vi "NPSV FIFO test.vi"() -> ()   [LabVIEW 2019]
uses:
  Reverse Polarity.ctl
  Forward Polarity.ctl
  Motion Controller Slot.ctl
  Stepper Output Configuration.ctl
  Axis Select.ctl
  MsgTypeDef.ctl
  DataDef.ctl
  <vilib>/NI/Modbus Library/API/Modbus API.lvclass
  <vilib>/WPC Systems Ltd/GECO Driver/Lib/GECOBase/GECO_Driver Class/GECO_Driver.lvclass
  <vilib>/WPC Systems Ltd/GECO Driver/Lib/GECOMotion/GECOMotion/_typedefine/Axis Select.ctl
  <vilib>/WPC Systems Ltd/GECO Driver/Lib/GECOBase/GECO_Driver Class/Motion/_typedefine/GECO_Stepper Output Configuration.ctl
  <vilib>/WPC Systems Ltd/GECO Driver/Lib/GECOBase/GECO_Driver Class/Motion/_typedefine/GECO_Motion Operation Mode.ctl
  <vilib>/WPC Systems Ltd/GECO Driver/Lib/GECOBase/GECO_Driver Class/GECO_SlotName.ctl
  <vilib>/WPC Systems Ltd/GECO Driver/Lib/GECOBase/GECO_Driver Class/Motion/_typedefine/GECO_ActiveHighLow.ctl
  <vilib>/WPC Systems Ltd/GECO Driver/Lib/GECOMotion/GECOMotion/GECO Motion.lvclass
  GyroDef.ctl
  <vilib>/Instr/_visa.llb/VISA Configure Serial Port (Instr).vi
panel:
  out "error IO 2":errorcluster
  out "error IO":errorcluster
  out "實際角度":cluster{"A":dbl, "B":dbl}={"A"=-3.299667554384925, "B"=3.520332445615068}
  out "實際角度Chart":cluster{"X":dbl, "Y":dbl}(graph)={"X"=-3.299667554384925, "Y"=3.520332445615068} caption="Waveform Chart - dark"
  out "Gyro\nPeriod":u32
  in  "Main Setting Tab":T1(tab)
  in  "TimerON":bool
  in  "Timer(ms)":i32=1
  in  "Serial Port":refnum<visa-resource-name>="COM3"
  in  "TCP slave port":u32=1
  in  "baud rate":u32=115200
  in  "Byte bits":u32=8
  in  "Modbus Address Starting":u32
  in  "Modbus Number of Inputs":u32=10000
  in  "Resource Name":tag="rio://192.168.0.224/RIO0"
  in  "Servo on":bool
  in  "Axis Select":T2
  in  "Stepper Output Configuration":T3=enum."CW/CCW(Two Pulse)"
  in  "Forward Enable?":bool=TRUE
  in  "Reverse Enable?":bool=TRUE
  in  "Motion Operation Mode":T4(ring)=enum."Velocity"
  in  "Forward Polarity":T5
  in  "Reverse Polarity":T6
  in  "Motion Controller Slot":T7
  in  "Target Position (0)":dbl=10000.0
  in  "Acceleration (100000)":u32=300000
  in  "Velocity (10000)":dbl=100000.0
  in  "Deacceleration (100000)":u32=300000
  in  "PID gains setting Tab":enum32{"Axis 1", "Axis 2", "Axis 3"}(tab)
  in  "PID gains":T8={"proportional gain (Kc)"=0.75, "integral time (Ti, min)"=0.01, "derivative time (Td, min)"=0.0} {"derivative time (Td, min)" format="%#_3f"; "integral time (Ti, min)" format="%#_3f"; "proportional gain (Kc)" format="%#_3f"}
  in  "PID gains 2":T8={"proportional gain (Kc)"=0.75, "integral time (Ti, min)"=0.01, "derivative time (Td, min)"=0.0} {"derivative time (Td, min)" format="%#_3f"; "integral time (Ti, min)" format="%#_3f"; "proportional gain (Kc)" format="%#_3f"}
  in  "PID gains 3":T8={"proportional gain (Kc)"=0.75, "integral time (Ti, min)"=0.01, "derivative time (Td, min)"=0.0} {"derivative time (Td, min)" format="%#_3f"; "integral time (Ti, min)" format="%#_3f"; "proportional gain (Kc)" format="%#_3f"}
  in  "ZABStop":bool
  in  "B":i32
  in  "A":i32
  in  "Z":i32=50
  in  "ZAB Start":bool
  in  "Move Setting":T9
  out "Axis 1":T10
  out "Axis 2":T10
  out "Axis 3":T10
  out "RT error out":errorcluster
  out "Program Period":u32
  out "RT Program Period":u32
  in  "ServoButtonControl":T11
  in  "Connect":bool
  in  "Close":bool
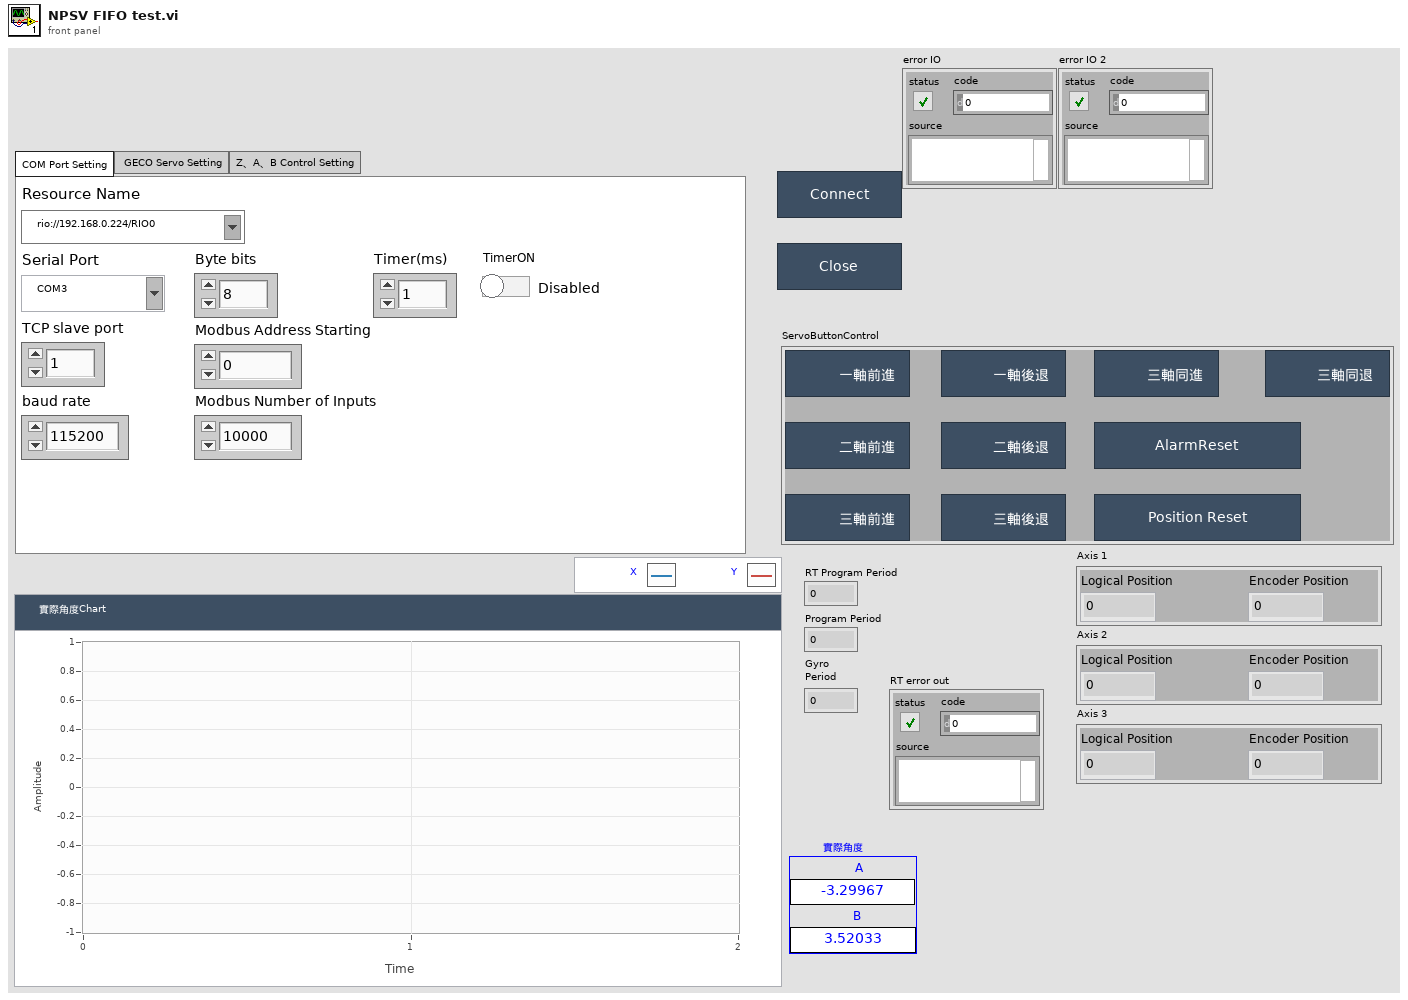
[diagram p1: front panel]
types:
  T1 = enum32{"COM Port Setting", " GECO Servo Setting", "Z、A、B Control Setting"}
  T2 = typedef "Axis Select.ctl" = enum16{"Axis 1", "Axis 2", "Axis 3", "Axis 4"}
  T3 = typedef "Stepper Output Configuration.ctl" = enum16{"Step/Dir(One Pulse)", "CW/CCW(Two Pulse)"}
  T4 = enum16{"Absolute Position", "Relative Position", "Velocity"}
  T5 = typedef "Forward Polarity.ctl" = enum16{"Active High", "Active Low"}
  T6 = typedef "Reverse Polarity.ctl" = enum16{"Active High", "Active Low"}
  T7 = typedef "Motion Controller Slot.ctl" = enum16{"C1", "C2", "C3", "C4"}
  T8 = cluster{"proportional gain (Kc)":dbl, "integral time (Ti, min)":dbl, "derivative time (Td, min)":dbl}
  T9 = typedef "軌跡設定.ctl" = u16
  T10 = cluster{"Encoder Position":i32, "Logical Position":i32}
  T11 = cluster{"三軸同退":bool, "三軸同進":bool, "三軸後退":bool, "三軸前進":bool, "二軸後退":bool, "二軸前進":bool, "一軸後退":bool, "一軸前進":bool, "Reset Encoder Position":bool, "AlarmReset":bool}
  T12 = typedef "GyroDef.ctl" = cluster{"Byte bits":u16, "baud rate":u32, "實際角度":cluster{"A":dbl, "B":dbl}, "COM Port":refnum<visa-resource-name>, "Save Path":refnum<file>}
  T13 = typedef "DataDef.ctl" = cluster{"address starting":u16, "狀態":enum16{"初始化", "讀取", "寫入", "停止"}, "理想角度":cluster{"A":dbl, "B":dbl}, "register values":i16[], "Modbus COM":refnum<class "Modbus API.lvclass">, "TCP slave port":u16, " baud rate":u32, "Byte bits":u16, "ServoButtonControl":cluster{"三軸同退":bool, "三軸同進":bool, "三軸後退":bool, "三軸前進":bool, "二軸後退":bool, "二軸前進":bool, "一軸後退":bool, "一軸前進":bool}, "Serial Number":string, "GECO_Driver out":refnum<class "GECO_Driver.lvclass">, "number of inputs":u16, "ServoSetting":cluster{"Axis Select":T14, "Stepper Output Configuration":T15, "Motion Operation Mode":T16, "Motion Controller Slot":T17, "Singel Axis Move Paramters":cluster{"Motion Operation Mode":T16, "Target Position (0)":i32, "Velocity (10000)":i32, "Acceleration (100000)":u32, "Deacceleration (100000)":u32}, "Reverse":cluster{"Reverse Enable":bool, "Reverse Polarity":T18}, "Forward":cluster{"Forward Enable":bool, "Forward Polarity":T18}}, "GECO Motion out":refnum<class "GECO Motion.lvclass">, "Servo on":bool, "Axis 1 Position":cluster{"Encoder Position":i32, "Logical Position":i32}, "Axis 2 Position":cluster{"Encoder Position":i32, "Logical Position":i32}, "Axis 3 Position":cluster{"Encoder Position":i32, "Logical Position":i32}, "PIDSetting":cluster{"Z":i32, "A":i32, "B":i32, "Move Setting":T19, "Axis Pulse":dbl, "Axis Length":dbl, "PID gains ":cluster{"proportional gain (Kc)":dbl, "integral time (Ti, min)":dbl, "derivative time (Td, min)":dbl}}, "resource name":tag, "Save Path":refnum<file>}
  T14 = typedef "GECO Motion.lvclass/Axis Select.ctl" = enum16{"Axis 1", "Axis 2", "Axis 3", "Axis 4"}
  T15 = typedef "GECO_Driver.lvclass/GECO_Stepper Output Configuration.ctl" = enum16{"Step/Dir(One Pulse)", "CW/CCW(Two Pulse)"}
  T16 = typedef "GECO_Driver.lvclass/GECO_Motion Operation Mode.ctl" = enum16{"Absolute Position", "Relative Position", "Velocity"}
  T17 = typedef "GECO_Driver.lvclass/GECO_SlotName.ctl" = enum16{"C1", "C2", "C3", "C4"}
  T18 = typedef "GECO_Driver.lvclass/GECO_ActiveHighLow.ctl" = enum16{"Active High", "Active Low"}
  T19 = typedef "­y¸ñ.ctl" = u16
  T20 = typedef "MsgTypeDef.ctl" = cluster{"CMD":string, "DATA":variant}
  T21 = enum16{"open", "replace", "create", "open or create", "replace or create", "replace or create with confirmation"}
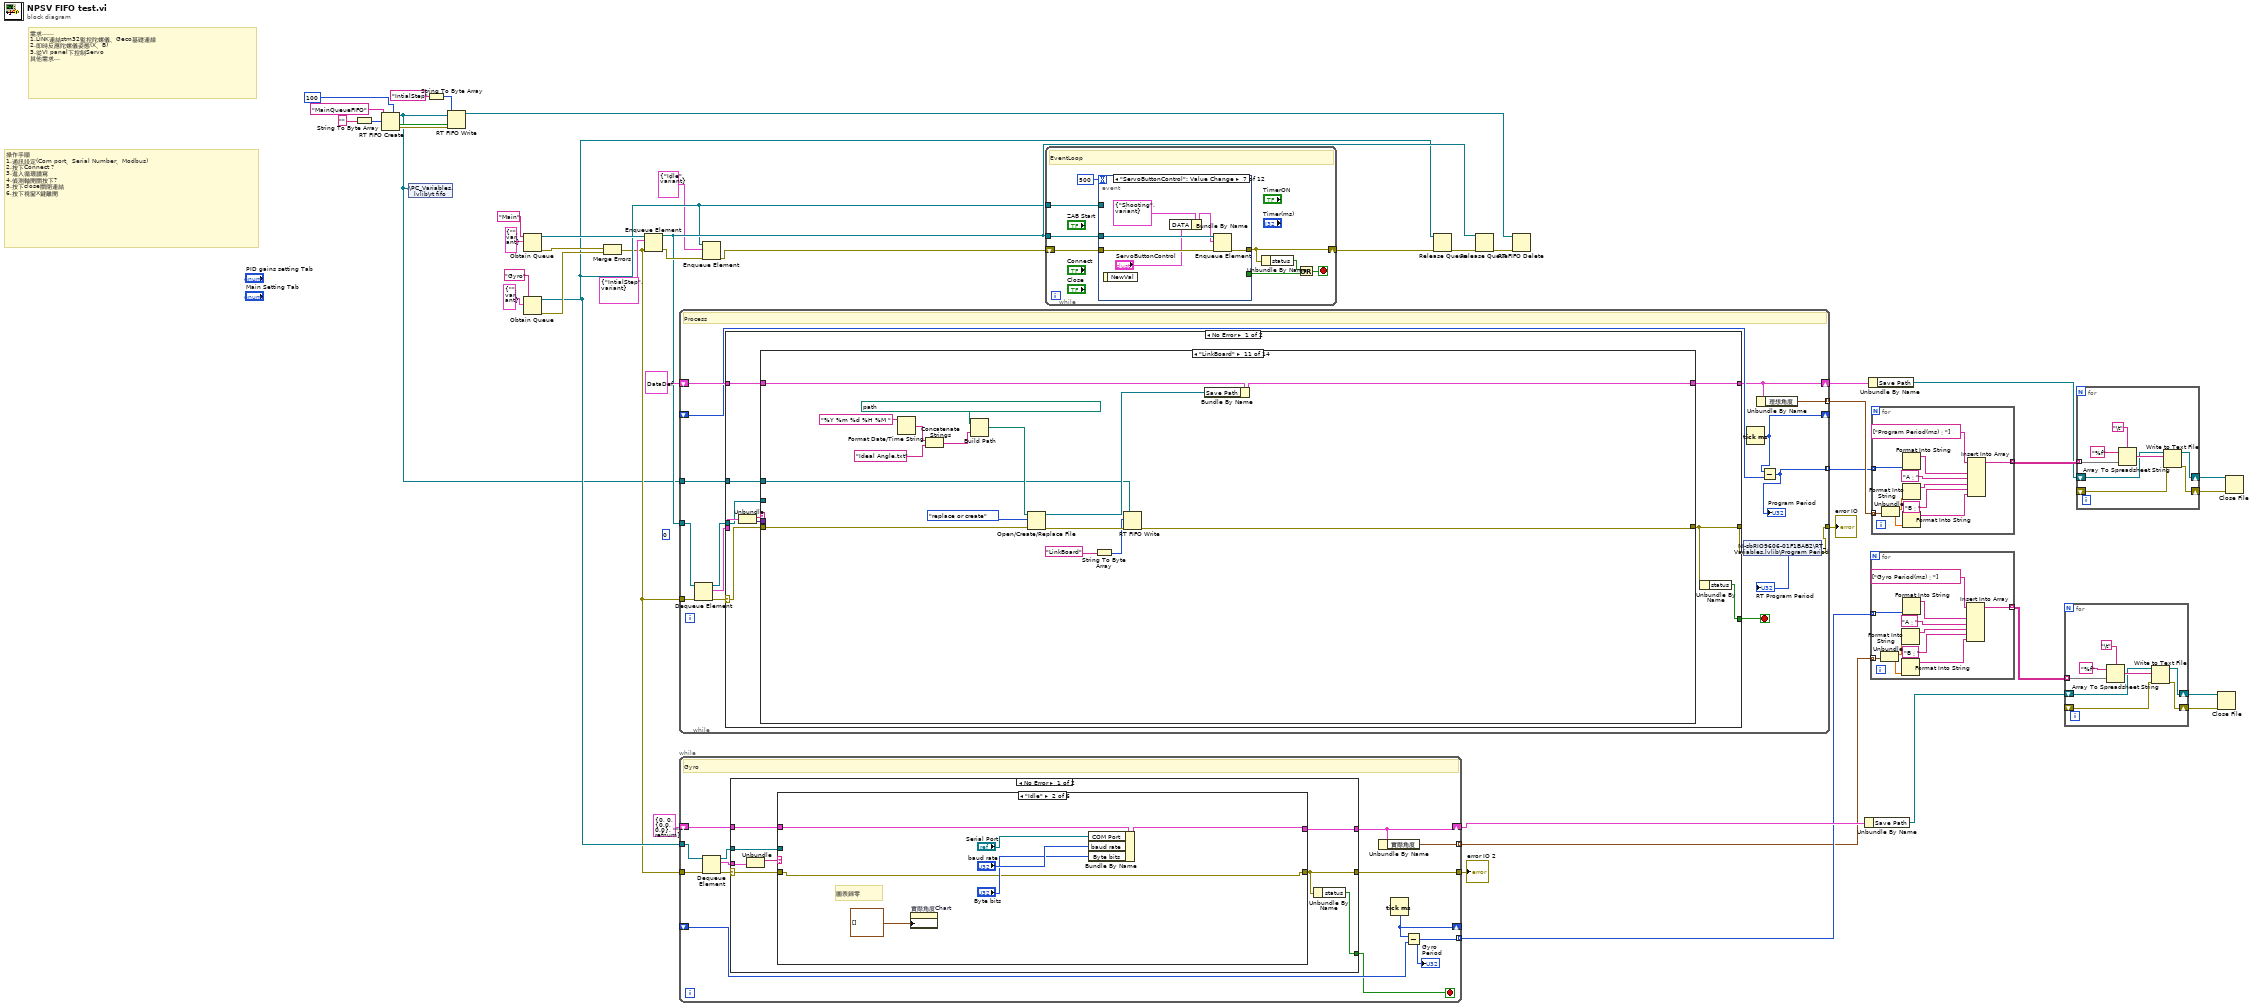
[diagram p0: block diagram]
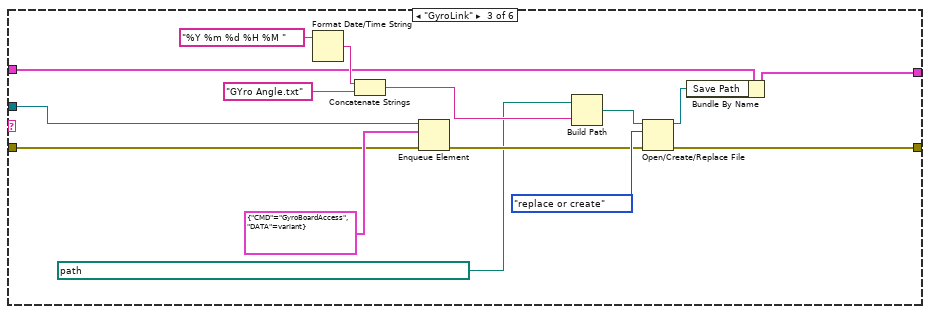
[diagram p3: hidden frame]
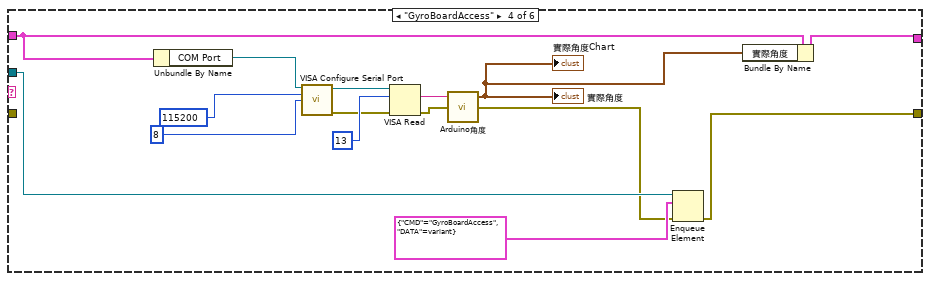
[diagram p4: hidden frame]
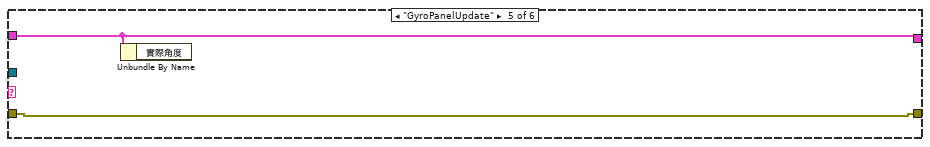
[diagram p5: hidden frame]
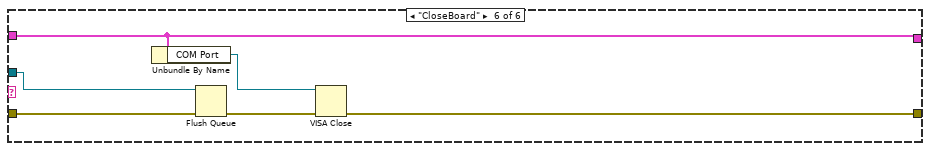
[diagram p6: hidden frame]
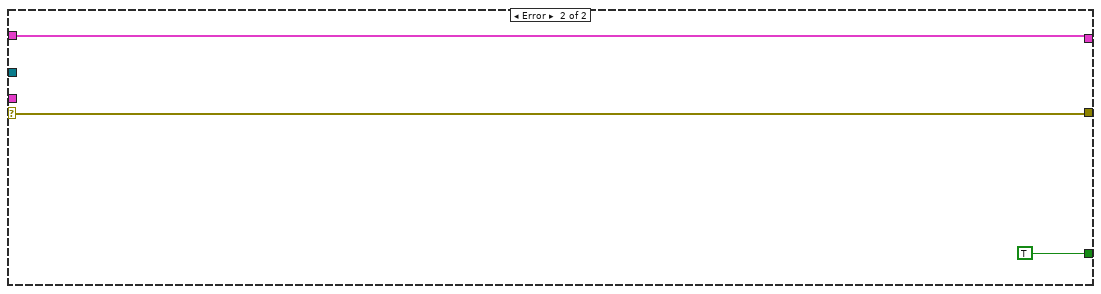
[diagram p7: hidden frame]
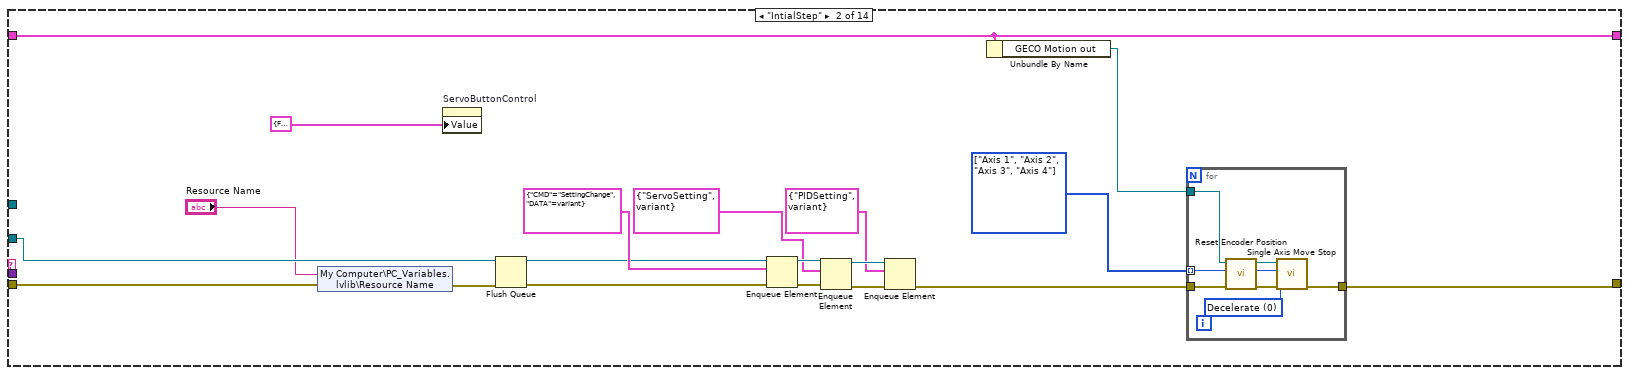
[diagram p9: hidden frame]
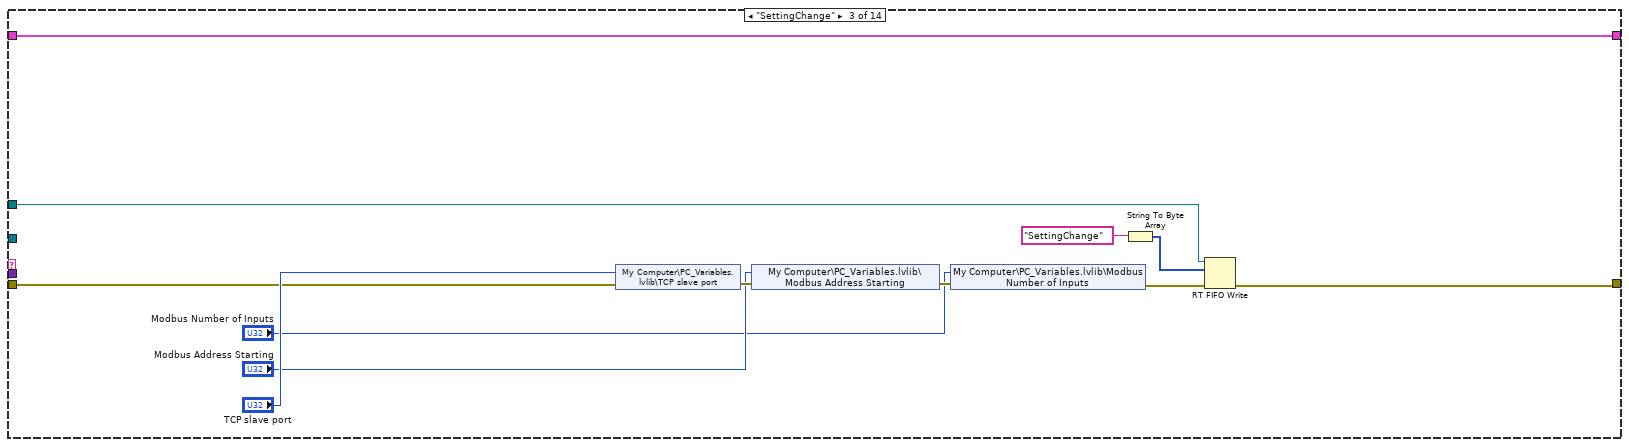
[diagram p10: hidden frame]
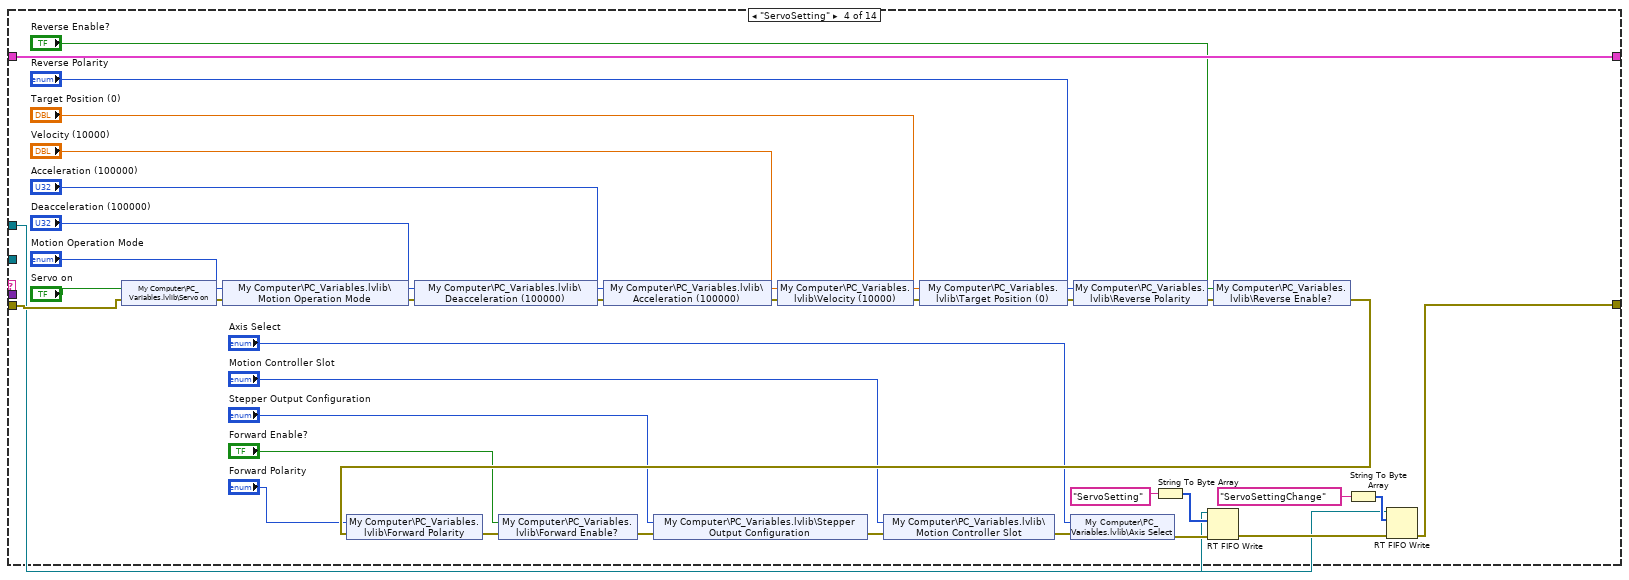
[diagram p11: hidden frame]
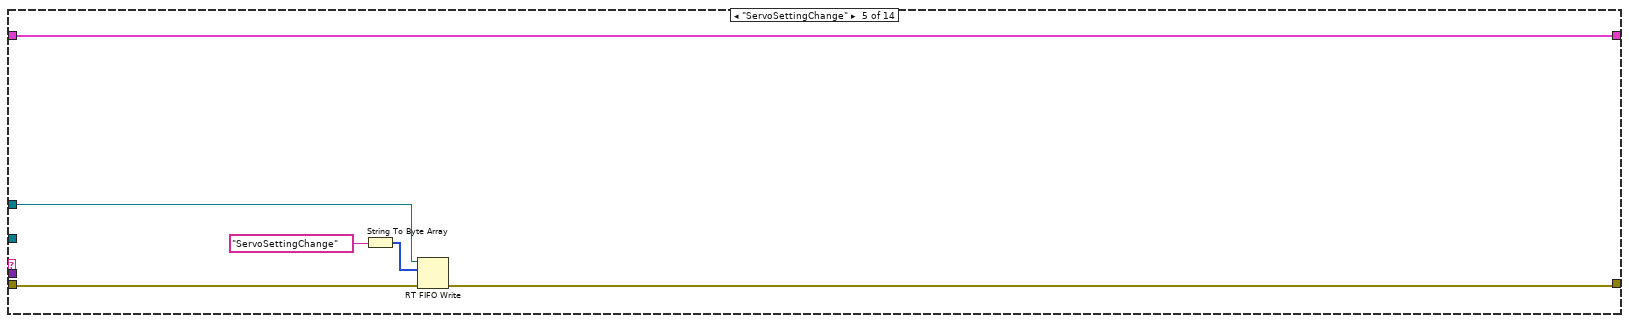
[diagram p12: hidden frame]
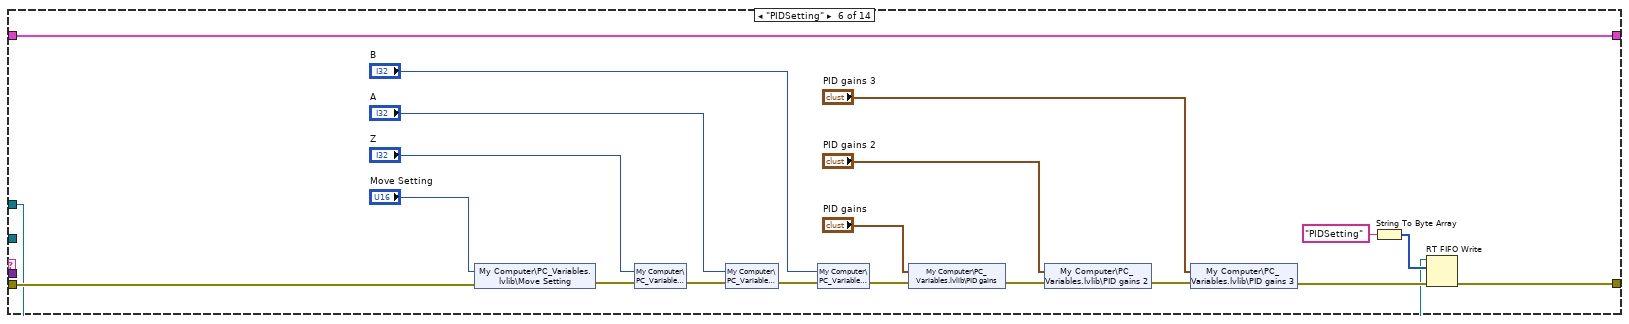
[diagram p13: hidden frame]
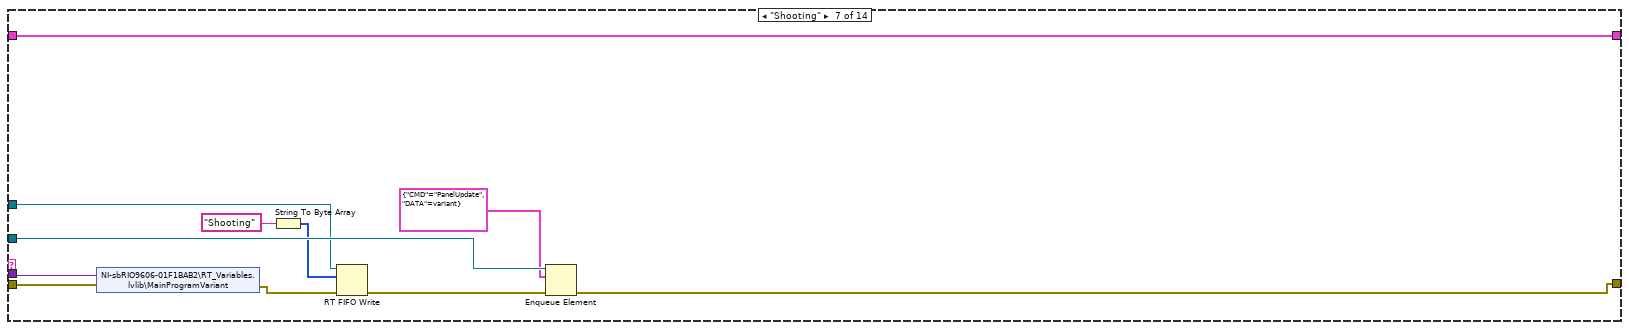
[diagram p14: hidden frame]
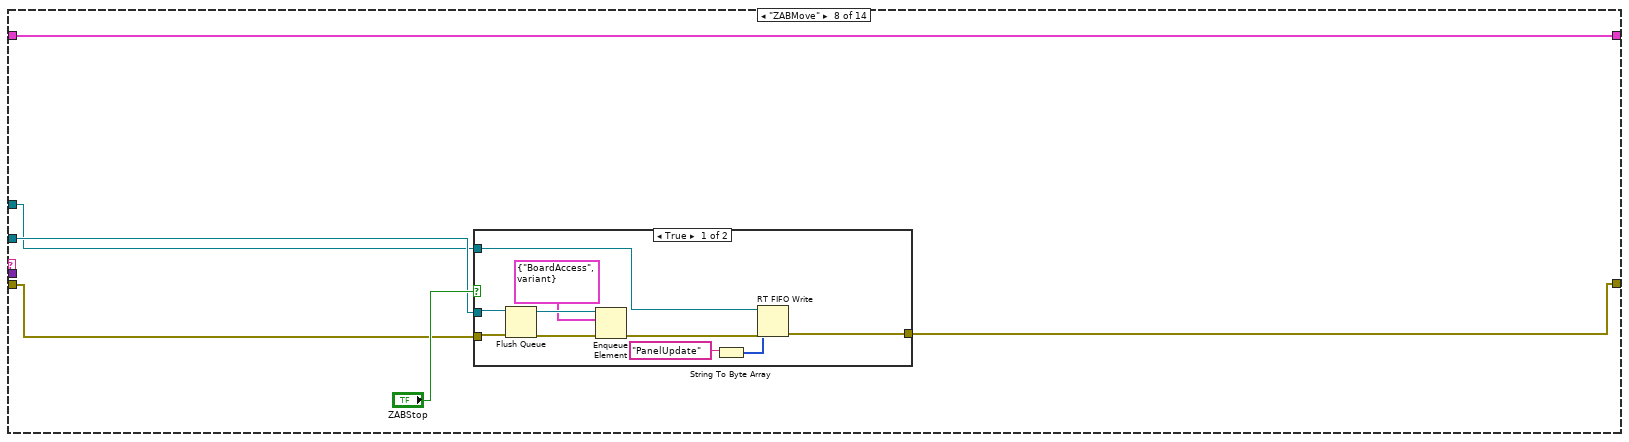
[diagram p15: hidden frame]
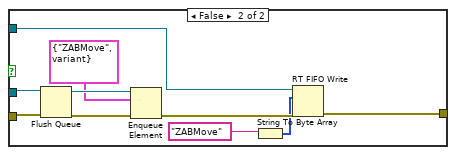
[diagram p16: hidden frame]
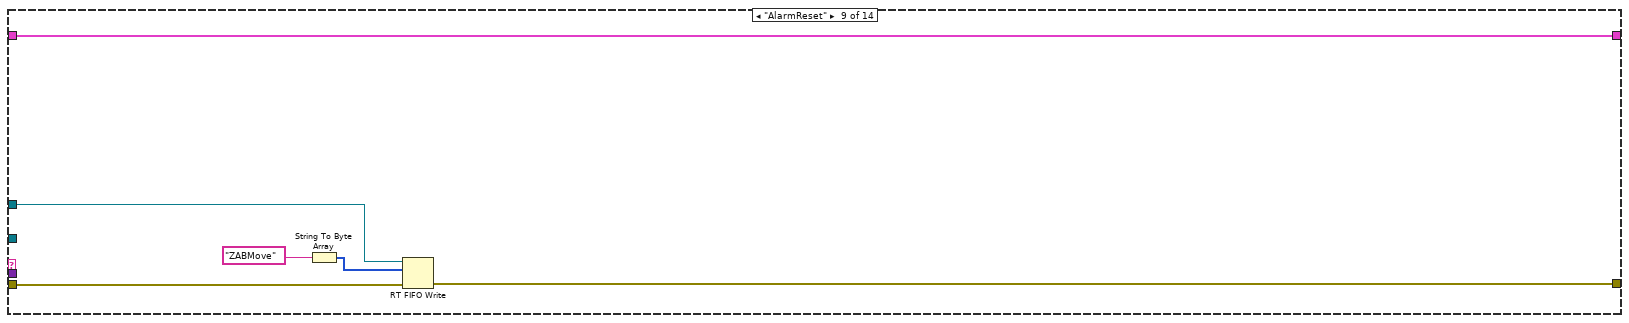
[diagram p17: hidden frame]
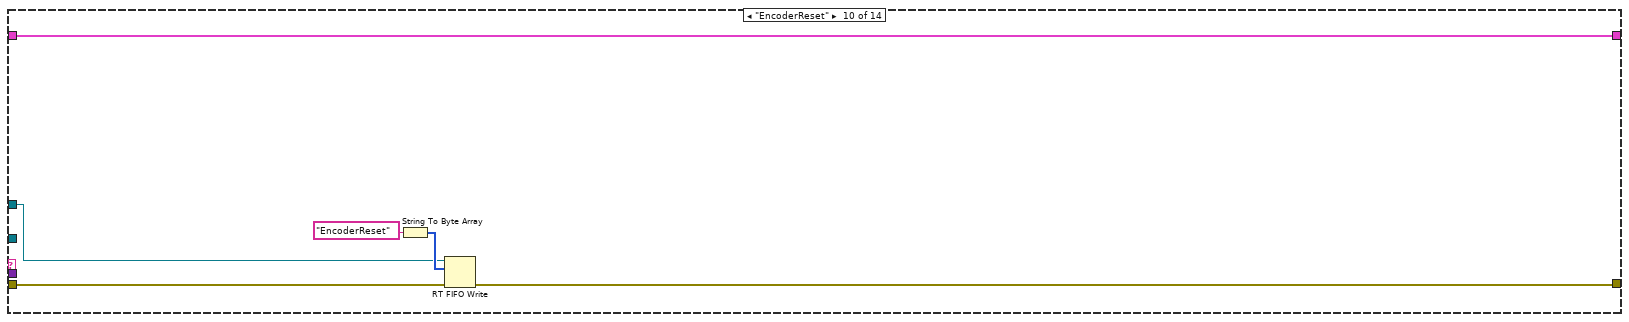
[diagram p18: hidden frame]
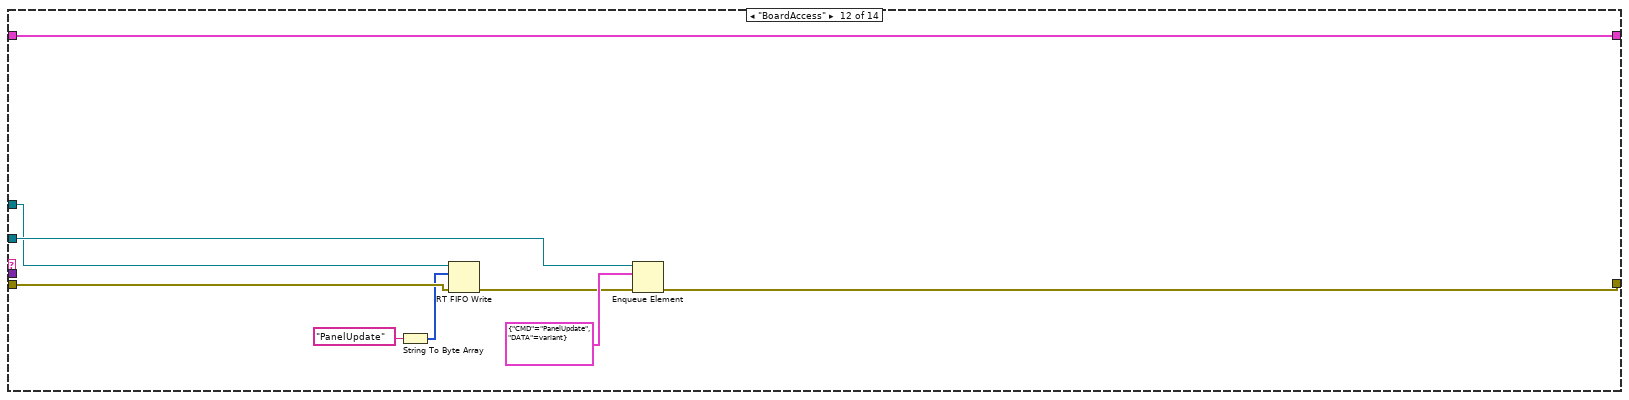
[diagram p19: hidden frame]
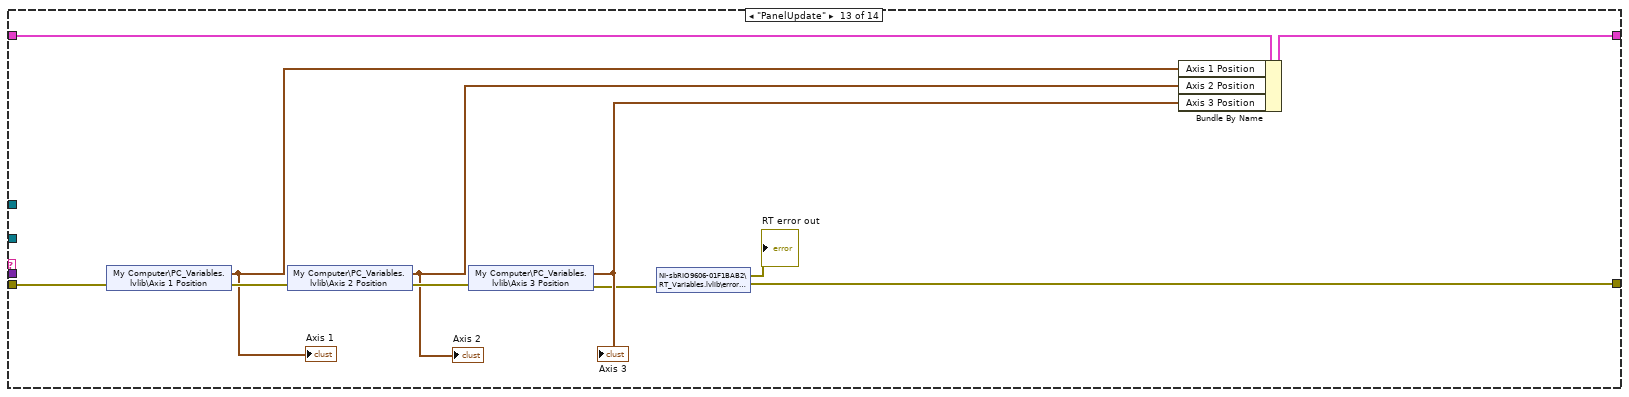
[diagram p20: hidden frame]
diagram:
  (unwired) 0
  # "操作手順\n1.通訊設定(Com port、Serial Number、Modbus)\n2.按下Connect ?\n3.進入循環讀寫\n4.偵測軸開關按下?\n5.按下close關閉連結\n6.按下視窗X鍵離開"
  # "需求......\n1.LINK連結stm32監控陀螺儀、Geco基礎連線\n2.即時反應陀螺儀姿態(X、B)\n3.從VI panel下控制Servo\n其他需求..."
  n1 = String To Byte Array(string="") -> (unsigned byte array=w11:u8[])
  n2 = RT FIFO Create(0:"MainQueueFIFO" ("name (unnamed)"), 1:w11, 6:u32 100 ("elements in array (1)")) -> (8:w3:refnum<k33>, 10:w8:bool, 11:w9:errorcluster)  [unwired: 5 in]
  n3 = shared-variable ".\\PC_Variables.lvlib\\rt fifo"(w3) -> ()  [unwired: 1 in, 1 out]
  n4 = String To Byte Array(string="IntialStep" ("CMD")) -> (unsigned byte array=w6:u8[])
  n5 = RT FIFO Write(0:w3, 1:w6, 3:w9, 5:w8) -> (8:w4:refnum<k33>)  [unwired: 1 in, 3 out]
  n6 = Obtain Queue(name (unnamed)="Main", element data type=T20 {"CMD"="", "DATA"=variant}) -> (queue out=w41:refnum<queue>, error out=w36:errorcluster)  [unwired: 3 in, 1 out]
  n7 = Obtain Queue(name (unnamed)="Gyro", element data type=T20 {"CMD"="", "DATA"=variant}) -> (queue out=w31:refnum<queue>, error out=w37:errorcluster)  [unwired: 3 in, 1 out]
  n8 = Merge Errors(w36, w37) -> (w29:errorcluster)
  n9 = Enqueue Element(queue=w41, element=T20 {"CMD"="IntialStep", "DATA"=variant}, error in (no error)=w29) -> (queue out=w32:refnum<queue>, error out=w34:errorcluster)  [unwired: 1 in, 1 out]
  n10 = while {
    tunnel: w32 -> [w61]
    shift-right: [w52] -> w24
    shift-left: T13 {"address starting"=0, "狀態"=enum."初始化", "理想角度"={"A"=0.0, "B"=0.0}, "register values"=[], "Modbus COM"=refnum, "TCP slave port"=1, " baud rate"=0, "Byte bits"=0, "ServoButtonControl"={"三軸同退"=FALSE, "三軸同進"=FALSE, "三軸後退"=FALSE, "三軸前進"=FALSE, "二軸後退"=FALSE, "二軸前進"=FALSE, "一軸後退"=FALSE, "一軸前進"=FALSE}, "Serial Number"="", "GECO_Driver out"=refnum, "number of inputs"=0, "ServoSetting"={"Axis Select"=enum."Axis 1", "Stepper Output Configuration"=enum."Step/Dir(One Pulse)", "Motion Operation Mode"=enum."Absolute Position", "Motion Controller Slot"=enum."C1", "Singel Axis Move Paramters"={"Motion Operation Mode"=enum."Velocity", "Target Position (0)"=10000, "Velocity (10000)"=1, "Acceleration (100000)"=100000, "Deacceleration (100000)"=1}, "Reverse"={"Reverse Enable"=FALSE, "Reverse Polarity"=enum."Active Low"}, "Forward"={"Forward Enable"=FALSE, "Forward Polarity"=enum."Active Low"}}, "GECO Motion out"=refnum, "Servo on"=FALSE, "Axis 1 Position"={"Encoder Position"=0, "Logical Position"=0}, "Axis 2 Position"={"Encoder Position"=0, "Logical Position"=0}, "Axis 3 Position"={"Encoder Position"=0, "Logical Position"=0}, "PIDSetting"={"Z"=10000, "A"=10000, "B"=10000, "Move Setting"=1, "Axis Pulse"=10000.0, "Axis Length"=10000.0, "PID gains "={"proportional gain (Kc)"=1.0, "integral time (Ti, min)"=0.01, "derivative time (Td, min)"=0.0}}, "resource name"="", "Save Path"=refnum} -> [w57]
    tunnel: w29 -> [w55]
    shift-right: [w54] -> _
    shift-left: _ -> [w53]
    tunnel: [w51] -> w27 mode=indexing
    tunnel: [w50] -> w26 mode=indexing
    tunnel: [w48] -> w13
    tunnel: w3 -> [w46]
    stop <- w58 stop-if-true
    # "Process"
    n11 = Dequeue Element(queue=w61, error in (no error)=w55) -> (queue out=w56:refnum<queue>, element=w59:T20, error out=w60:errorcluster)  [unwired: 1 in, 1 out]
    n12 = case shown="No Error" w60 {
      selector: w60 -> [w67 w267]
      tunnel: w59 -> [w71 _]
      tunnel: [w64 TRUE] -> w58
      tunnel: [w69 w268] -> w52
      tunnel: w57 -> [w68 w268]
      tunnel: w56 -> [w66 _]
      tunnel: [w63 w267] -> w49
      tunnel: w46 -> [w62 _]
      frame No Error {
        n13 = Unbundle(w71) -> ("CMD"=w70:string, "DATA"=w65:variant)
        n14 = case shown="\"LinkBoard\"" w70 {
          tunnel: [w73 w77 w112 w147 w153 w173 w184 w186 w216 w222 w229 w244 w257 w266] -> w69
          tunnel: w68 -> [w73 w77 w112 w147 w153 w173 w184 w186 w216 w222 w238 w244 w258 w266]
          tunnel: w67 -> [w72 w76 w106 w146 w152 w172 w180 w188 w215 w221 w232 w242 w254 w264]
          tunnel: [w72 w87 w104 w114 w151 w157 w182 w187 w213 w217 w223 w246 w248 w259] -> w63
          tunnel: w66 -> [_ w81 _ _ _ _ w183 w189 _ _ _ w247 _ w265]
          tunnel: w65 -> [_ _ _ _ _ _ w179 _ _ _ _ _ _ _]
          tunnel: w62 -> [_ _ w101 w113 w148 w154 w175 w185 w211 w218 w226 w241 _ w260]
          frame Default {
          }
          frame "IntialStep" {
            w85 = T14[] [enum."Axis 1", enum."Axis 2", enum."Axis 3", enum."Axis 4"] items=["Axis 1", "Axis 2", "Axis 3", "Axis 4"]
            n15 = shared-variable "My Computer\\PC_Variables.lvlib\\Resource Name"("Resource Name", error in=w76) -> (error out=w74:errorcluster)
            n16 = property on="ServoButtonControl" class="Clust"("Value"=T11 {"三軸同退"=FALSE, "三軸同進"=FALSE, "三軸後退"=FALSE, "三軸前進"=FALSE, "二軸後退"=FALSE, "二軸前進"=FALSE, "一軸後退"=FALSE, "一軸前進"=FALSE, "Reset Encoder Position"=FALSE, "AlarmReset"=FALSE} ("ServoButtonControl")) -> ()  [unwired: 2 in, 2 out]
            n17 = Flush Queue(queue=w81, error in (no error)=w74) -> (queue out=w80:refnum<queue>, error out=w79:errorcluster)  [unwired: 1 out]
            n18 = Enqueue Element(queue=w80, element=T20 {"CMD"="SettingChange", "DATA"=variant}, error in (no error)=w79) -> (queue out=w90:refnum<queue>, error out=w91:errorcluster)  [unwired: 1 in, 1 out]
            n19 = Enqueue Element(queue=w90, element=T20 {"CMD"="ServoSetting", "DATA"=variant}, error in (no error)=w91) -> (queue out=w84:refnum<queue>, error out=w83:errorcluster)  [unwired: 1 in, 1 out]
            n20 = Enqueue Element(queue=w84, element=T20 {"CMD"="PIDSetting", "DATA"=variant}, error in (no error)=w83) -> (error out=w78:errorcluster)  [unwired: 1 in, 2 out]
            n21 = Unbundle By Name(w77) -> ("GECO Motion out"=w86:refnum<class "GECO Motion.lvclass">)
            n22 = for {
              tunnel: w78 -> [w100]
              tunnel: [w94] -> w87
              tunnel: w86 -> [w99]
              tunnel: w85 -> [w98] mode=indexing
              w93 = u16 0 items=["Decelerate", "Halt"] ("Motion Stop Type")
              n23 = call <vilib>:"Reset Encoder Position.vi"("error in (no error)"=w100, "Axis Select"=w98, "GECO Motion in"=w99) -> ("error out"=w97:errorcluster, "Axis Select out"=w96:T14, "GECO Motion out"=w95:refnum<class "GECO Motion.lvclass">)  [unwired: 6 in]
              n24 = call <vilib>:"Single Axis Move Stop.vi"("error in (no error)"=w97, "Motion Stop Type"=w93, "Axis Select"=w96, "GECO Motion in"=w95) -> ("error out"=w94:errorcluster)  [unwired: 5 in, 2 out]
            }
          }
          frame "SettingChange" {
            n25 = shared-variable "My Computer\\PC_Variables.lvlib\\TCP slave port"("TCP slave port", error in=w106) -> (error out=w111:errorcluster)
            n26 = shared-variable "My Computer\\PC_Variables.lvlib\\Modbus Address Starting"("Modbus Address Starting", error in=w111) -> (error out=w110:errorcluster)
            n27 = shared-variable "My Computer\\PC_Variables.lvlib\\Modbus Number of Inputs"("Modbus Number of Inputs", error in=w110) -> (error out=w105:errorcluster)
            n28 = String To Byte Array(string="SettingChange" ("CMD")) -> (unsigned byte array=w102:u8[])
            n29 = RT FIFO Write(0:w101, 1:w102, 3:w105) -> (11:w104:errorcluster)  [unwired: 2 in, 3 out]
          }
          frame "ServoSetting" {
            n30 = shared-variable "My Computer\\PC_Variables.lvlib\\Servo on"("Servo on", error in=w146) -> (error out=w144:errorcluster)
            n31 = shared-variable "My Computer\\PC_Variables.lvlib\\Motion Operation Mode"("Motion Operation Mode", error in=w144) -> (error out=w143:errorcluster)
            n32 = shared-variable "My Computer\\PC_Variables.lvlib\\Deacceleration (100000)"("Deacceleration (100000)", error in=w143) -> (error out=w142:errorcluster)
            n33 = shared-variable "My Computer\\PC_Variables.lvlib\\Acceleration (100000)"("Acceleration (100000)", error in=w142) -> (error out=w141:errorcluster)
            n34 = shared-variable "My Computer\\PC_Variables.lvlib\\Velocity (10000)"("Velocity (10000)", error in=w141) -> (error out=w140:errorcluster)
            n35 = shared-variable "My Computer\\PC_Variables.lvlib\\Target Position (0)"("Target Position (0)", error in=w140) -> (error out=w139:errorcluster)
            n36 = shared-variable "My Computer\\PC_Variables.lvlib\\Reverse Polarity"("Reverse Polarity", error in=w139) -> (error out=w138:errorcluster)
            n37 = String To Byte Array(string="ServoSetting" ("CMD")) -> (unsigned byte array=w117:u8[])
            n38 = shared-variable "My Computer\\PC_Variables.lvlib\\Reverse Enable?"("Reverse Enable?", error in=w138) -> (error out=w145:errorcluster)
            n39 = shared-variable "My Computer\\PC_Variables.lvlib\\Forward Polarity"("Forward Polarity", error in=w145) -> (error out=w129:errorcluster)
            n40 = shared-variable "My Computer\\PC_Variables.lvlib\\Forward Enable?"("Forward Enable?", error in=w129) -> (error out=w128:errorcluster)
            n41 = shared-variable "My Computer\\PC_Variables.lvlib\\Stepper Output Configuration"("Stepper Output Configuration", error in=w128) -> (error out=w127:errorcluster)
            n42 = shared-variable "My Computer\\PC_Variables.lvlib\\Motion Controller Slot"("Motion Controller Slot", error in=w127) -> (error out=w126:errorcluster)
            n43 = shared-variable "My Computer\\PC_Variables.lvlib\\Axis Select"("Axis Select", error in=w126) -> (error out=w119:errorcluster)
            n44 = RT FIFO Write(0:w113, 1:w117, 3:w119) -> (11:w115:errorcluster)  [unwired: 2 in, 3 out]
            n45 = String To Byte Array(string="ServoSettingChange" ("CMD")) -> (unsigned byte array=w116:u8[])
            n46 = RT FIFO Write(0:w113, 1:w116, 3:w115) -> (11:w114:errorcluster)  [unwired: 2 in, 3 out]
          }
          frame "ServoSettingChange" {
            n47 = String To Byte Array(string="ServoSettingChange" ("CMD")) -> (unsigned byte array=w149:u8[])
            n48 = RT FIFO Write(0:w148, 1:w149, 3:w152) -> (11:w151:errorcluster)  [unwired: 2 in, 3 out]
          }
          frame "PIDSetting" {
            n49 = shared-variable "My Computer\\PC_Variables.lvlib\\Move Setting"("Move Setting", error in=w172) -> (error out=w171:errorcluster)
            n50 = shared-variable "My Computer\\PC_Variables.lvlib\\Z"("Z", error in=w171) -> (error out=w170:errorcluster)
            n51 = shared-variable "My Computer\\PC_Variables.lvlib\\A"("A", error in=w170) -> (error out=w169:errorcluster)
            n52 = shared-variable "My Computer\\PC_Variables.lvlib\\B"("B", error in=w169) -> (error out=w161:errorcluster)
            n53 = shared-variable "My Computer\\PC_Variables.lvlib\\PID gains"("PID gains", error in=w161) -> (error out=w160:errorcluster)
            n54 = shared-variable "My Computer\\PC_Variables.lvlib\\PID gains 2"("PID gains 2", error in=w160) -> (error out=w159:errorcluster)
            n55 = shared-variable "My Computer\\PC_Variables.lvlib\\PID gains 3"("PID gains 3", error in=w159) -> (error out=w158:errorcluster)
            n56 = String To Byte Array(string="PIDSetting" ("CMD")) -> (unsigned byte array=w155:u8[])
            n57 = RT FIFO Write(0:w154, 1:w155, 3:w158) -> (11:w157:errorcluster)  [unwired: 2 in, 3 out]
          }
          frame "Shooting" {
            n58 = shared-variable "NI-sbRIO9606-01F1BAB2\\RT_Variables.lvlib\\MainProgramVariant"(w179, error in=w180) -> (error out=w178:errorcluster)
            n59 = String To Byte Array(string="Shooting" ("CMD")) -> (unsigned byte array=w174:u8[])
            n60 = RT FIFO Write(0:w175, 1:w174, 3:w178) -> (11:w177:errorcluster)  [unwired: 2 in, 3 out]
            n61 = Enqueue Element(queue=w183, element=T20 {"CMD"="PanelUpdate", "DATA"=variant}, error in (no error)=w177) -> (error out=w182:errorcluster)  [unwired: 1 in, 2 out]
          }
          frame "ZABMove" {
            n62 = case shown="True" "ZABStop" {
              tunnel: [w194 w204] -> w187
              tunnel: w189 -> [w197 w207]
              tunnel: w188 -> [w196 w206]
              tunnel: w185 -> [w191 w201]
              frame True {
                n63 = Flush Queue(queue=w197, error in (no error)=w196) -> (queue out=w200:refnum<queue>, error out=w199:errorcluster)  [unwired: 1 out]
                n64 = Enqueue Element(queue=w200, element=T20 {"CMD"="BoardAccess", "DATA"=variant}, error in (no error)=w199) -> (error out=w195:errorcluster)  [unwired: 1 in, 2 out]
                n65 = String To Byte Array(string="PanelUpdate" ("CMD")) -> (unsigned byte array=w193:u8[])
                n66 = RT FIFO Write(0:w191, 1:w193, 3:w195) -> (11:w194:errorcluster)  [unwired: 2 in, 3 out]
              }
              frame False {
                n67 = Flush Queue(queue=w207, error in (no error)=w206) -> (queue out=w210:refnum<queue>, error out=w209:errorcluster)  [unwired: 1 out]
                n68 = Enqueue Element(queue=w210, element=T20 {"CMD"="ZABMove", "DATA"=variant}, error in (no error)=w209) -> (error out=w205:errorcluster)  [unwired: 1 in, 2 out]
                n69 = String To Byte Array(string="ZABMove" ("CMD")) -> (unsigned byte array=w203:u8[])
                n70 = RT FIFO Write(0:w201, 1:w203, 3:w205) -> (11:w204:errorcluster)  [unwired: 2 in, 3 out]
              }
            }
          }
          frame "AlarmReset" {
            n71 = String To Byte Array(string="ZABMove" ("CMD")) -> (unsigned byte array=w212:u8[])
            n72 = RT FIFO Write(0:w211, 1:w212, 3:w215) -> (11:w213:errorcluster)  [unwired: 2 in, 3 out]
          }
          frame "EncoderReset" {
            n73 = String To Byte Array(string="EncoderReset" ("CMD")) -> (unsigned byte array=w219:u8[])
            n74 = RT FIFO Write(0:w218, 1:w219, 3:w221) -> (11:w217:errorcluster)  [unwired: 2 in, 3 out]
          }
          frame "LinkBoard" {
            n75 = Format Date/Time String(time format string (%c)="%Y %m %d %H %M ") -> (date/time string=w236:string)  [unwired: 2 in]
            n76 = Concatenate Strings(w236, "Ideal Angle.txt" ("element")) -> (w235:string)
            n77 = Build Path(base path=path "C:/Users/baby3/OneDrive/Desktop/碩論/陀螺儀監控平台控制/GyroData", name or relative path=w235) -> (appended path=w230:path)
            n78 = Open/Create/Replace File(file path (use dialog)=w230, error in=w232, operation (0:open)=T21."replace or create") -> (refnum out=w228:refnum<file>, error out=w227:errorcluster)  [unwired: 3 in, 1 out]
            n79 = String To Byte Array(string="LinkBoard" ("CMD")) -> (unsigned byte array=w225:u8[])
            n80 = RT FIFO Write(0:w226, 1:w225, 3:w227) -> (11:w223:errorcluster)  [unwired: 2 in, 3 out]
            n81 = Bundle By Name(cluster=w238, "Save Path"=w228) -> (w229:T13)
          }
          frame "BoardAccess" {
            n82 = String To Byte Array(string="PanelUpdate" ("CMD")) -> (unsigned byte array=w240:u8[])
            n83 = RT FIFO Write(0:w241, 1:w240, 3:w242) -> (11:w243:errorcluster)  [unwired: 2 in, 3 out]
            n84 = Enqueue Element(queue=w247, element=T20 {"CMD"="PanelUpdate", "DATA"=variant}, error in (no error)=w243) -> (error out=w246:errorcluster)  [unwired: 1 in, 2 out]
          }
          frame "PanelUpdate" {
            n85 = shared-variable "My Computer\\PC_Variables.lvlib\\Axis 1 Position"(error in=w254) -> (w253:T10, error out=w256:errorcluster)
            "Axis 1" <- w253
            n86 = shared-variable "My Computer\\PC_Variables.lvlib\\Axis 2 Position"(error in=w256) -> (w252:T10, error out=w255:errorcluster)
            "Axis 2" <- w252
            n87 = shared-variable "My Computer\\PC_Variables.lvlib\\Axis 3 Position"(error in=w255) -> (w251:T10, error out=w249:errorcluster)
            "Axis 3" <- w251
            n88 = shared-variable "NI-sbRIO9606-01F1BAB2\\RT_Variables.lvlib\\error out"(error in=w249) -> (→"RT error out":errorcluster, error out=w248:errorcluster)
            n89 = Bundle By Name(cluster=w258, "Axis 1 Position"=w253, "Axis 2 Position"=w252, "Axis 3 Position"=w251) -> (w257:T13)
          }
          frame "CloseBoard" {
            n90 = Flush Queue(queue=w265, error in (no error)=w264) -> (error out=w263:errorcluster)  [unwired: 2 out]
            n91 = String To Byte Array(string="CloseBoard" ("CMD")) -> (unsigned byte array=w262:u8[])
            n92 = RT FIFO Write(0:w260, 1:w262, 3:w263) -> (11:w259:errorcluster)  [unwired: 2 in, 3 out]
          }
        }
        n93 = Unbundle By Name(w63) -> ("status"=w64:bool)
      }
      frame Error {
      }
    }
    n94 = shared-variable "NI-sbRIO9606-01F1BAB2\\RT_Variables.lvlib\\Program Period"(error in=w49) -> (→"RT Program Period":u32, error out=w48:errorcluster)
    n95 = Tick Count (ms)() -> (millisecond timer value=w54:u32)
    n96 = Unbundle By Name(w52) -> ("理想角度"=w51:cluster{"A":dbl, "B":dbl})
    n97 = Subtract(x=w54, y=w53) -> (x-y=w50:u32)
    "Program Period" <- w50
  }
  "error IO" <- w13
  n98 = while {
    tunnel: w31 -> [w282]
    tunnel: w29 -> [w281]
    shift-right: [w276] -> w22
    shift-left: T12 {"Byte bits"=0, "baud rate"=0, "實際角度"={"A"=0.0, "B"=0.0}, "COM Port"="", "Save Path"=refnum} -> [w277]
    tunnel: [w275] -> w15 mode=indexing
    shift-right: [w274] -> _
    shift-left: _ -> [w273]
    tunnel: [w271] -> w12
    tunnel: [w270] -> w16 mode=indexing
    stop <- w272 stop-if-true
    # "Gyro"
    n99 = Dequeue Element(queue=w282, error in (no error)=w281) -> (queue out=w279:refnum<queue>, element=w278:T20, error out=w280:errorcluster)  [unwired: 1 in, 1 out]
    n100 = case shown="No Error" w280 {
      selector: w280 -> [w286 w338]
      tunnel: w279 -> [w285 _]
      tunnel: w278 -> [w290 _]
      tunnel: [w284 TRUE] -> w272
      tunnel: w277 -> [w288 w339]
      tunnel: [w287 w339] -> w276
      tunnel: [w283 w338] -> w271
      frame No Error {
        n101 = Unbundle(w290) -> ("CMD"=w289:string)  [unwired: 1 out]
        n102 = case shown="\"Idle\"" w289 {
          tunnel: [w292 w298 w303 w316 w331 w333] -> w287
          tunnel: w288 -> [w292 w299 w300 w326 w331 w333]
          tunnel: w286 -> [w291 w294 w306 _ w330 w337]
          tunnel: [w291 w294 w304 w322 w330 w334] -> w283
          tunnel: w285 -> [_ _ w313 w325 _ w335]
          frame Default {
          }
          frame "Idle" {
            # "圖表歸零"
            n103 = property on="實際角度Chart" class="WFChart (strict)"("History Data"=cluster{"X":dbl, "Y":dbl}[] []) -> ()  [unwired: 2 in, 2 out]
            n104 = Bundle By Name(cluster=w299, "COM Port"="Serial Port", "baud rate"="baud rate", "Byte bits"="Byte bits") -> (w298:T12)
          }
          frame "GyroLink" {
            n105 = Format Date/Time String(time format string (%c)="%Y %m %d %H %M ") -> (date/time string=w311:string)  [unwired: 2 in]
            n106 = Concatenate Strings(w311, "GYro Angle.txt" ("element")) -> (w308:string)
            n107 = Enqueue Element(queue=w313, element=T20 {"CMD"="GyroBoardAccess", "DATA"=variant}, error in (no error)=w306) -> (error out=w305:errorcluster)  [unwired: 1 in, 2 out]
            n108 = Build Path(base path=path "C:/Users/baby3/OneDrive/Desktop/碩論/陀螺儀監控平台控制/GyroData", name or relative path=w308) -> (appended path=w307:path)
            n109 = Open/Create/Replace File(file path (use dialog)=w307, error in=w305, operation (0:open)=T21."replace or create") -> (refnum out=w302:refnum<file>, error out=w304:errorcluster)  [unwired: 3 in, 1 out]
            n110 = Bundle By Name(cluster=w300, "Save Path"=w302) -> (w303:T12)
          }
          frame "GyroBoardAccess" {
            n111 = Unbundle By Name(w326) -> ("COM Port"=w319:refnum<visa-resource-name>)
            n112 = call-poly "VISA Configure Serial Port"("VISA resource name"=w319, "baud rate (9600)"=u32 115200, "data bits (8)"=u16 8) -> ("VISA resource name out"=w318:refnum<visa-resource-name>, "error out"=w317:errorcluster)  [unwired: 11 in]
            n113 = VISA Read(VISA resource name=w318, byte count=u32 13, error in (no error)=w317) -> (read buffer=w329:string, error out=w328:errorcluster)  [unwired: 2 out]
            n114 = call "Arduino角度.vi"("error in"=w328, "read buffer"=w329) -> ("error out"=w323:errorcluster, "Waveform Chart"=w315:cluster{dbl, dbl})  [unwired: 2 in]
            "實際角度" <- w315
            "實際角度Chart" <- w315
            n115 = Enqueue Element(queue=w325, element=T20 {"CMD"="GyroBoardAccess", "DATA"=variant}, error in (no error)=w323) -> (error out=w322:errorcluster)  [unwired: 1 in, 2 out]
            n116 = Bundle By Name(cluster=w326, "實際角度"=w315) -> (w316:T12)
          }
          frame "GyroPanelUpdate" {
            n117 = Unbundle By Name(w331) -> ()  [unwired: 1 out]
          }
          frame "CloseBoard" {
            n118 = Unbundle By Name(w333) -> ("COM Port"=w332:refnum<visa-resource-name>)
            n119 = Flush Queue(queue=w335, error in (no error)=w337) -> (error out=w336:errorcluster)  [unwired: 2 out]
            n120 = VISA Close(VISA resource name=w332, error in (no error)=w336) -> (error out=w334:errorcluster)
          }
        }
        n121 = Unbundle By Name(w283) -> ("status"=w284:bool)
      }
      frame Error {
      }
    }
    n122 = Unbundle By Name(w276) -> ("實際角度"=w275:cluster{"A":dbl, "B":dbl})
    n123 = Tick Count (ms)() -> (millisecond timer value=w274:u32)
    n124 = Subtract(x=w274, y=w273) -> (x-y=w270:u32)
    "Gyro\nPeriod" <- w270
  }
  "error IO 2" <- w12
  n125 = Enqueue Element(queue=w31, element=T20 {"CMD"="Idle", "DATA"=variant}, error in (no error)=w34) -> (error out=w33:errorcluster)  [unwired: 1 in, 2 out]
  n126 = while {
    shift-right: [w344] -> w45
    shift-left: w33 -> [w347]
    tunnel: w32 -> [w348]
    tunnel: w31 -> [w342]
    stop <- w345 stop-if-true
    # "EventLoop"
    n127 = event shown="[6] \"ServoButtonControl\": Value Change" {
      selector: _ -> [_ _ _ _ _ _ _ _ _ _ _ _]
      dyn-events: _ -> [_ _ _ _ _ _ _ _ _ _ _ _]
      timeout: 500 -> [_ _ _ _ _ _ _ _ _ _ _ _]
      tunnel: w348 -> [w352 w356 w360 w367 w371 w375 w381 w385 _ w393 w401 w404]
      tunnel: w347 -> [w351 w355 w359 w366 w370 w374 w380 w384 w391 w395 w400 w406]
      tunnel: [w350 w354 w358 w363 w369 w373 w379 w383 w390 w394 w398 w403] -> w344
      tunnel: [_ _ _ _ _ _ _ _ _ _ _ w408] -> w346
      tunnel: w342 -> [_ _ _ w361 _ _ _ _ w388 _ w396 w407]
      event "Modbus Number of Inputs", "Serial Port", "TCP slave port", "baud rate", "Byte bits", "Modbus Address Starting": Value Change {
        n128 = event-data() -> ()  [unwired: 1 in, 1 out]
        n129 = Enqueue Element(queue=w352, element=T20 {"CMD"="SettingChange", "DATA"=variant}, error in (no error)=w351) -> (error out=w350:errorcluster)  [unwired: 1 in, 2 out]
      }
      event "Forward Enable?", "Reverse Enable?", "Motion Operation Mode", "Target Position (0)", "Acceleration (100000)", "Velocity (10000)", "Deacceleration (100000)", "Servo on": Value Change {
        n130 = event-data() -> ()  [unwired: 1 in, 1 out]
        n131 = Enqueue Element(queue=w356, element=T20 {"CMD"="ServoSetting", "DATA"=variant}, error in (no error)=w355) -> (error out=w354:errorcluster)  [unwired: 1 in, 2 out]
      }
      event "Z", "A", "B": Value Change {
        n132 = event-data() -> ()  [unwired: 1 in, 2 out]
        n133 = Enqueue Element(queue=w360, element=T20 {"CMD"="PIDSetting", "DATA"=variant}, error in (no error)=w359) -> (error out=w358:errorcluster)  [unwired: 1 in, 2 out]
      }
      event "Connect": Value Change {
        n134 = event-data() -> ()  [unwired: 1 in, 1 out]
        n135 = Enqueue Element(queue=w367, element=T20 {"CMD"="LinkBoard", "DATA"=variant}, error in (no error)=w366) -> (error out=w364:errorcluster)  [unwired: 1 in, 2 out]
        n136 = Enqueue Element(queue=w361, element=T20 {"CMD"="GyroLink", "DATA"=variant}, error in (no error)=w364) -> (error out=w363:errorcluster)  [unwired: 1 in, 2 out]
      }
      event "ServoButtonControl.AlarmReset": Value Change {
        n137 = event-data() -> ()  [unwired: 1 in, 1 out]
        n138 = Enqueue Element(queue=w371, element=T20 {"CMD"="AlarmReset", "DATA"=variant}, error in (no error)=w370) -> (error out=w369:errorcluster)  [unwired: 1 in, 2 out]
      }
      event "ServoButtonControl.Reset Encoder Position": Value Change {
        n139 = event-data() -> ()  [unwired: 1 in, 1 out]
        n140 = Enqueue Element(queue=w375, element=T20 {"CMD"="EncoderReset", "DATA"=variant}, error in (no error)=w374) -> (error out=w373:errorcluster)  [unwired: 1 in, 2 out]
      }
      event "ServoButtonControl": Value Change {
        n141 = event-data() -> ()  [unwired: 1 in, 1 out]
        n142 = Bundle By Name(cluster=T20 {"CMD"="Shooting", "DATA"=variant} ("element"), "DATA"="ServoButtonControl") -> (w377:T20)
        n143 = Enqueue Element(queue=w381, element=w377, error in (no error)=w380) -> (error out=w379:errorcluster)  [unwired: 1 in, 2 out]
      }
      event "ZABStop", "ZAB Start": Value Change {
        n144 = event-data() -> ()  [unwired: 1 in, 2 out]
        n145 = Enqueue Element(queue=w385, element=T20 {"CMD"="ZABMove", "DATA"=variant}, error in (no error)=w384) -> (error out=w383:errorcluster)  [unwired: 1 in, 2 out]
      }
      event "TimerON": Value Change {
        n146 = event-data() -> ("NewVal"=w386:bool)  [unwired: 1 in]
        n147 = Bundle By Name(cluster=T20 {"CMD"="ChangeTimerState", "DATA"=variant} ("element"), "DATA"=w386) -> (w387:T20)
        n148 = Enqueue Element(queue=w388, element=w387, error in (no error)=w391) -> (error out=w390:errorcluster)  [unwired: 1 in, 2 out]
      }
      event Timeout {
        n149 = event-data() -> ()  [unwired: 1 in, 2 out]
        n150 = Enqueue Element(queue=w393, element=T20 {"CMD"="BoardAccess", "DATA"=variant}, error in (no error)=w395) -> (error out=w394:errorcluster)  [unwired: 1 in, 2 out]
      }
      event "Close": Value Change {
        w397 = T20 {"CMD"="CloseBoard", "DATA"=variant} ("element")
        n151 = event-data() -> ()  [unwired: 1 in, 1 out]
        n152 = Enqueue Element At Opposite End(queue=w401, element=w397, error in (no error)=w400) -> (error out=w399:errorcluster)  [unwired: 1 in, 2 out]
        n153 = Enqueue Element At Opposite End(queue=w396, element=w397, error in (no error)=w399) -> (error out=w398:errorcluster)  [unwired: 1 in, 2 out]
      }
      event Panel Close? {
        w402 = T20 {"CMD"="CloseBoard", "DATA"=variant} ("element")
        w408 = TRUE
        n154 = event-data() -> ()  [unwired: 1 in, 1 out]
        n155 = Enqueue Element At Opposite End(queue=w407, element=w402, error in (no error)=w406) -> (error out=w405:errorcluster)  [unwired: 1 in, 2 out]
        n156 = event-data("Discard?"=w408) -> ()  [unwired: 1 in, 1 out]
        n157 = Enqueue Element At Opposite End(queue=w404, element=w402, error in (no error)=w405) -> (error out=w403:errorcluster)  [unwired: 1 in, 2 out]
      }
    }
    n158 = Unbundle By Name(w344) -> ("status"=w343:bool)
    n159 = Or(x=w343, y=w346) -> (x .or. y?=w345:bool)
  }
  n160 = Release Queue(queue=w31, error in (no error)=w45) -> (error out=w35:errorcluster)  [unwired: 1 in, 2 out]
  n161 = Release Queue(queue=w32, error in (no error)=w35) -> (error out=w5:errorcluster)  [unwired: 1 in, 2 out]
  n162 = RT FIFO Delete(0:w4, 3:w5) -> ()  [unwired: 1 in, 1 out]
  n163 = Unbundle By Name(w22) -> ("Save Path"=w21:refnum<file>)
  n164 = Unbundle By Name(w24) -> ("Save Path"=w23:refnum<file>)
  n165 = for {
    tunnel: [w418] -> w14 mode=indexing
    tunnel: w15 -> [w417] mode=indexing
    tunnel: w16 -> [w414] mode=indexing
    n166 = Unbundle(w417) -> ("A"=w416:dbl, "B"=w415:dbl)
    n167 = Format Into String(w416) -> (resulting string=w411:string)  [unwired: 3 in, 1 out]
    n168 = Format Into String(w415) -> (resulting string=w410:string)  [unwired: 3 in, 1 out]
    n169 = Format Into String(w414) -> (resulting string=w413:string)  [unwired: 3 in, 1 out]
    n170 = Insert Into Array(array=string[] ["Gyro Period(ms)："], new element #1=w413, new element #2="A：", new element #3=w411, new element #4="B：", new element #5=w410) -> (w418:string[])  [unwired: 1 in]
  }
  n171 = for {
    tunnel: [w429] -> w25 mode=indexing
    tunnel: w27 -> [w428] mode=indexing
    tunnel: w26 -> [w425] mode=indexing
    n172 = Unbundle(w428) -> ("A"=w427:dbl, "B"=w426:dbl)
    n173 = Format Into String(w427) -> (resulting string=w422:string)  [unwired: 3 in, 1 out]
    n174 = Format Into String(w426) -> (resulting string=w420:string)  [unwired: 3 in, 1 out]
    n175 = Format Into String(w425) -> (resulting string=w424:string)  [unwired: 3 in, 1 out]
    n176 = Insert Into Array(array=string[] ["Program Period(ms)："], new element #1=w424, new element #2="A：", new element #3=w422, new element #4="B：", new element #5=w420) -> (w429:string[])  [unwired: 1 in]
  }
  n177 = for {
    shift-right: [w433] -> w19
    shift-left: w21 -> [w435]
    shift-right: [w434] -> w20
    shift-left: _ -> [w432]
    tunnel: w14 -> [w431] mode=indexing
    n178 = Array To Spreadsheet String(delimiter (Tab)="\t", array=w431, 3:"%f" ("format string")) -> (spreadsheet string=w436:string)
    n179 = Write to Text File(file (use dialog)=w435, text=w436, error in=w432) -> (refnum out=w433:refnum<file>, error out=w434:errorcluster)  [unwired: 1 in, 1 out]
  }
  n180 = for {
    tunnel: w25 -> [w441] mode=indexing
    shift-right: [w439] -> w17
    shift-left: w23 -> [w443]
    shift-right: [w440] -> w18
    shift-left: _ -> [w442]
    n181 = Array To Spreadsheet String(delimiter (Tab)="\t", array=w441, 3:"%f" ("format string")) -> (spreadsheet string=w444:string)
    n182 = Write to Text File(file (use dialog)=w443, text=w444, error in=w442) -> (refnum out=w439:refnum<file>, error out=w440:errorcluster)  [unwired: 1 in, 1 out]
  }
  n183 = Close File(refnum=w19, error in=w20) -> ()  [unwired: 2 out]
  n184 = Close File(refnum=w17, error in=w18) -> ()  [unwired: 2 out]
